vi "LVDimInterface.dis_stop_serving.vi"(5 "error in (no error)":errorcluster) -> (19 "error out":errorcluster)   [LabVIEW 2014, in "LVDimInterface.lvlib"]
doc: "This routine can be called by the server program in order to stop being a DIM Server.\n\n\nHistory: 16-DEC-2005, Dietrich Beck\n\nCopyright (C)\nGesellschaft für Schwerionenforschung, GSI\nPlanckstr. 1\n64291 Darmstadt\nGermany\n\nContact: D.Beck@gsi.de \n\nThis program is free software; you can redistribute it and/or modify it under the terms of the \nGNU General Public License as published by the Free Software Foundation; either version 2 of the license, or (at your option) any later version.\n\nThis program is distributed in the hope that it will be useful, but WITHOUT ANY WARRANTY; without even the implied warranty of MERCHANTABILITY or FITNESS FOR A PARTICULAR PURPOSE. See the GNU General License for more details (http://www.gnu.org).\n\nGesellschaft für Schwerionenforschung, GSI\nPlanckstr. 1, 64291 Darmstadt, Germany\nFor all questions and ideas contact D. Beck.\nLast update: 16-DEC-2005"
uses:
  LVDimInterface.lvlib
  shs/packages/dmdriver/DMirrorPCS/libDimWrapper.dll
  bin/libDimWrapper.so
  bin/libDimWrapperSPL.dll
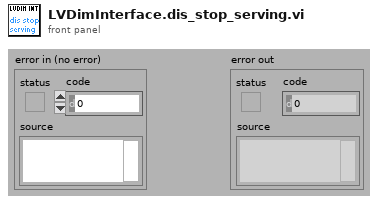
[diagram p1: front panel]
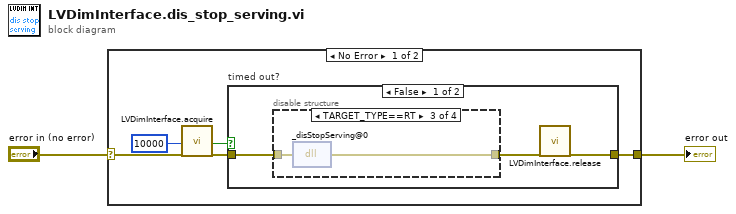
[diagram p0: block diagram]
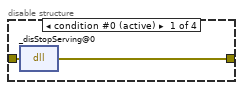
[diagram p2: hidden frame]
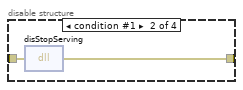
[diagram p3: hidden frame]
diagram:
  n1 = case shown="No Error" "error in (no error)" {
    selector: "error in (no error)" -> [w3 w19]
    tunnel: [w7 w19] -> w1
    frame No Error {
      n2 = call "LVDimInterface.acquire.vi"("ms timeout (10000)"=10000 ("ms timeout (-1)"), "error in (no error)"=w3) -> ("timed out"=w4:bool, "error out"=w6:errorcluster)  [unwired: 16 in]
      n3 = case "timed out?" shown="False" w4 {
        tunnel: [w9 w18] -> w7
        tunnel: w6 -> [w10 w18]
        frame False {
          n4 = disable-structure "Conditional Disable Structure" shown="TARGET_TYPE==RT" {
            disable-tunnel: w10 -> [w12 w13 w16 w17]
            disable-tunnel: [w11 w14 w15 w17] -> w8
            frame condition #0 (active) {
              n5 = dll-call lib="D:/Git/CS-framework/CSlibraries-extern/shs/packages/dmdriver/DMirrorPCS/libDimWrapper.dll" fn="_disStopServing@0" label="disStopServing"(error in=w12) -> (error out=w11:errorcluster)  [unwired: 3 in, 1 out]
            }
            frame condition #1 {
              n6 = dll-call lib="D:/Git/CS-framework/CSlibraries/DimLVEvent/bin/libDimWrapper.so" fn="disStopServing"(error in=w13) -> (error out=w14:errorcluster)  [unwired: 3 in, 1 out]
            }
            frame condition #2 {
              n7 = dll-call lib="D:/Git/CS-framework/CSlibraries/DimLVEvent/bin/libDimWrapperSPL.dll" fn="_disStopServing@0" label="libDimWrapper.so:disStopServing"(error in=w16) -> (error out=w15:errorcluster)  [unwired: 3 in, 1 out]
            }
            frame condition #3 {
            }
          }
          n8 = call "LVDimInterface.release.vi"("error in (no error)"=w8) -> ("error out"=w9:errorcluster)  [unwired: 18 in]
        }
        frame True {
        }
      }
    }
    frame Error {
    }
  }
  "error out" <- w1
